vi "摄像头.vi"() -> ()   [LabVIEW 2018]
uses:
  <vilib>/userdefined/High Color/IMAQdx.ctl
  <vilib>/vision/driver/NI_Vision_Acquisition_Software.lvlib
panel:
  out "Image":T1(plugin-control)
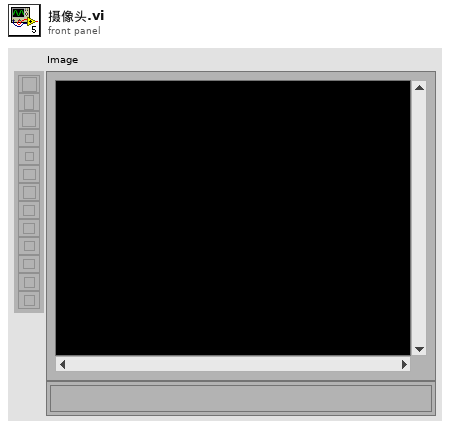
[diagram p1: front panel]
types:
  T1 = typedef "IMAQ Image.ctl" = refnum<image>
  T2 = typedef "IMAQdx.ctl" = refnum<k21>
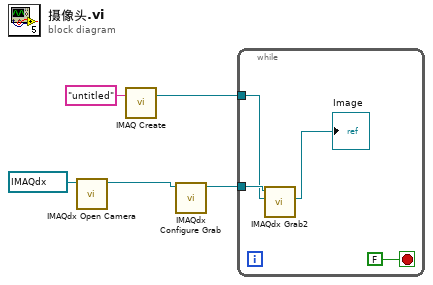
[diagram p0: block diagram]
diagram:
  n1 = call <vilib>:"IMAQdx Open Camera.vi"("Session In"=T2 "cam0") -> ("Session Out"=w4:T2)  [unwired: 9 in, 1 out]
  n2 = call "IMAQ Create"("Image Name"="untitled") -> ("New Image"=w2:T1)  [unwired: 4 in, 1 out]
  n3 = call <vilib>:"IMAQdx Configure Grab.vi"("Session In"=w4) -> ("Session Out"=w3:T2)  [unwired: 9 in, 1 out]
  n4 = while {
    tunnel: w3 -> [w8]
    tunnel: w2 -> [w6]
    stop <- FALSE stop-if-true
    n5 = call <vilib>:"IMAQdx Grab2.vi"("Image In"=w6, "Session In"=w8) -> ("Image Out"=→"Image":T1)  [unwired: 6 in, 3 out]
  }
